vi "YActor_SendUiEvent.vi"(6 "Event":string, 8 "ErrorIn":errorcluster, 9 "Data":variant, 11 "YActor in":refnum<class "YActor.lvclass">) -> (0 "ErrorOut":errorcluster, 3 "YActor out":refnum<class "YActor.lvclass">)   [LabVIEW 2021, in "YActor.lvclass"]
uses:
  YActor.lvclass
  YActor.lvclass/YActor.ctl
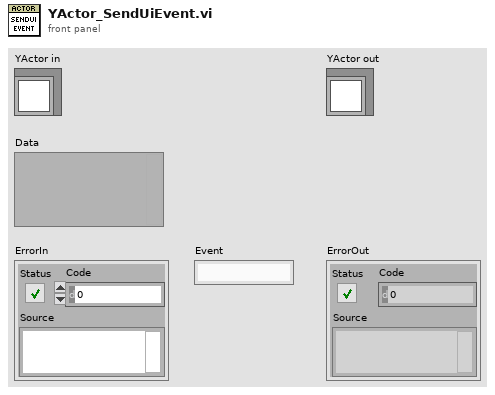
[diagram p1: front panel]
types:
  T1 = cluster{"UIEvent":cluster{"Event":string, "This":refnum<class>, "Data":variant}}
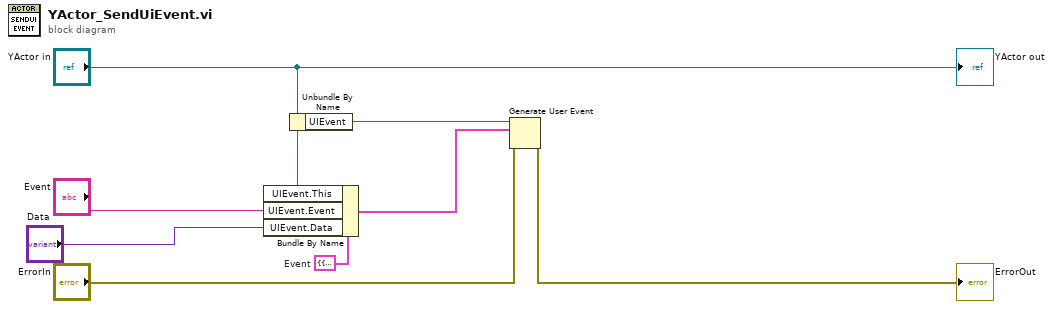
[diagram p0: block diagram]
diagram:
  w2 = T1 {"UIEvent"={"Event"="", "This"=refnum, "Data"=variant}}  # Event
  n1 = Bundle By Name(cluster=w2, "UIEvent.This"="YActor in", "UIEvent.Event"="Event", "UIEvent.Data"="Data") -> (w5:T1)
  n2 = Unbundle By Name("YActor in") -> ("UIEvent"=w8:refnum<user-event>)
  n3 = Generate User Event(user event=w8, event data cluster=w5, error in="ErrorIn") -> (error out=→"ErrorOut":errorcluster)  [unwired: 1 in, 1 out]
  "YActor out" <- "YActor in"
